vi "Create SearchMatch Queues.vi"(8 "error in (no error)":errorcluster) -> (0 "error out":errorcluster, 3 "Message Queues":T1)   [LabVIEW 2023, in "Front Panel Message Queue.lvlib"]
doc: "This VI creates and initializes all the message queues for your application. If your application requires more than one message queue, right-click the \"Message Queues\" constant above and select Open Type Def. Add the new Message Queue(s) to the type definition, then initialize them in this VI."
uses:
  Front Panel Message Queue.lvlib
  Calibrazione Message Queues.ctl
  Message Cluster.ctl
  SearchMatch Message Queues.ctl
  Enqueue Message (Single).vi
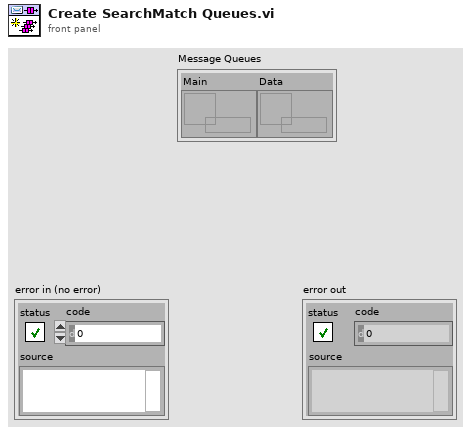
[diagram p1: front panel]
types:
  T1 = typedef "Front Panel Message Queue.lvlib/Calibrazione Message Queues.ctl" = cluster{"Main":refnum<queue>, "Data":refnum<queue>}
  T2 = typedef "Front Panel Message Queue.lvlib/SearchMatch Message Queues.ctl" = cluster{"Main":refnum<queue>, "Data":refnum<queue>}
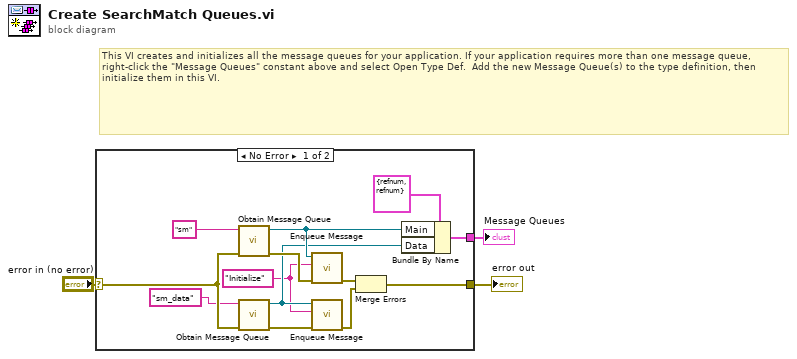
[diagram p0: block diagram]
diagram:
  # "This VI creates and initializes all the message queues for your application. If your application requires more than one message queue, right-click the \"Message Queues\" constant above and select Open Type Def.  Add the new Message Queue(s) to the type definition, then initialize them in this VI."
  n1 = case shown="No Error" "error in (no error)" {
    selector: "error in (no error)" -> [w8 w17]
    tunnel: [w11 w17] -> w3
    tunnel: [w16 _] -> w1
    frame No Error {
      w7 = "Initialize" ("Message")
      n2 = call "Obtain Message Queue.vi"("error in (no error)"=w8, "name"="sm") -> ("error out"=w15:errorcluster, "Message Queue"=w14:refnum<queue>)  [unwired: 8 in]
      n3 = call "Obtain Message Queue.vi"("error in (no error)"=w8, "name"="sm_data") -> ("error out"=w13:errorcluster, "Message Queue"=w12:refnum<queue>)  [unwired: 8 in]
      n4 = call-poly "Enqueue Message.vi"("error in (no error)"=w15, "Message"=w7, "Message Queue"=w14) -> ("error out"=w10:errorcluster)  [unwired: 7 in, 1 out]
      n5 = call-poly "Enqueue Message.vi"("error in (no error)"=w13, "Message"=w7, "Message Queue"=w12) -> ("error out"=w9:errorcluster)  [unwired: 7 in, 1 out]
      n6 = Merge Errors(w10, w9) -> (w11:errorcluster)
      n7 = Bundle By Name(cluster=T2 {"Main"=refnum, "Data"=refnum} ("Message Queues"), "Main"=w14, "Data"=w12) -> (w16:T2)
    }
    frame Error {
    }
  }
  "error out" <- w3
  "Message Queues" <- w1
